vi "Test Harness.vi"() -> ()   [LabVIEW 2014, in "Waveform-Processing-Custom-Device Engine.lvlib"]
uses:
  Waveform-Processing-Custom-Device Engine.lvlib
  <vilib>/NI Veristand/Custom Device API/Hardware Interface Driver VI Operation.ctl
  <vilib>/NI Veristand/Custom Device API/Custom Device Item Ref.ctl
  <vilib>/NI Veristand/Custom Device API/Custom Device API.lvlib
panel:
  in  "Data Queue Element":dbl[](array[numeric])
  in  "Loop Rate":u32
  in  "Stop":bool
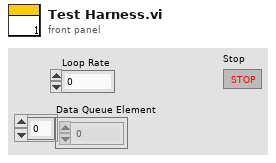
[diagram p1: front panel]
types:
  T1 = typedef "Custom Device API.lvlib/Hardware Interface Driver VI Operation.ctl" = enum16{"Initialize", "Start", "Read Data from HW", "Write Data to HW", "Close"}
  T2 = typedef "Custom Device API.lvlib/Custom Device Item Ref.ctl" = u64
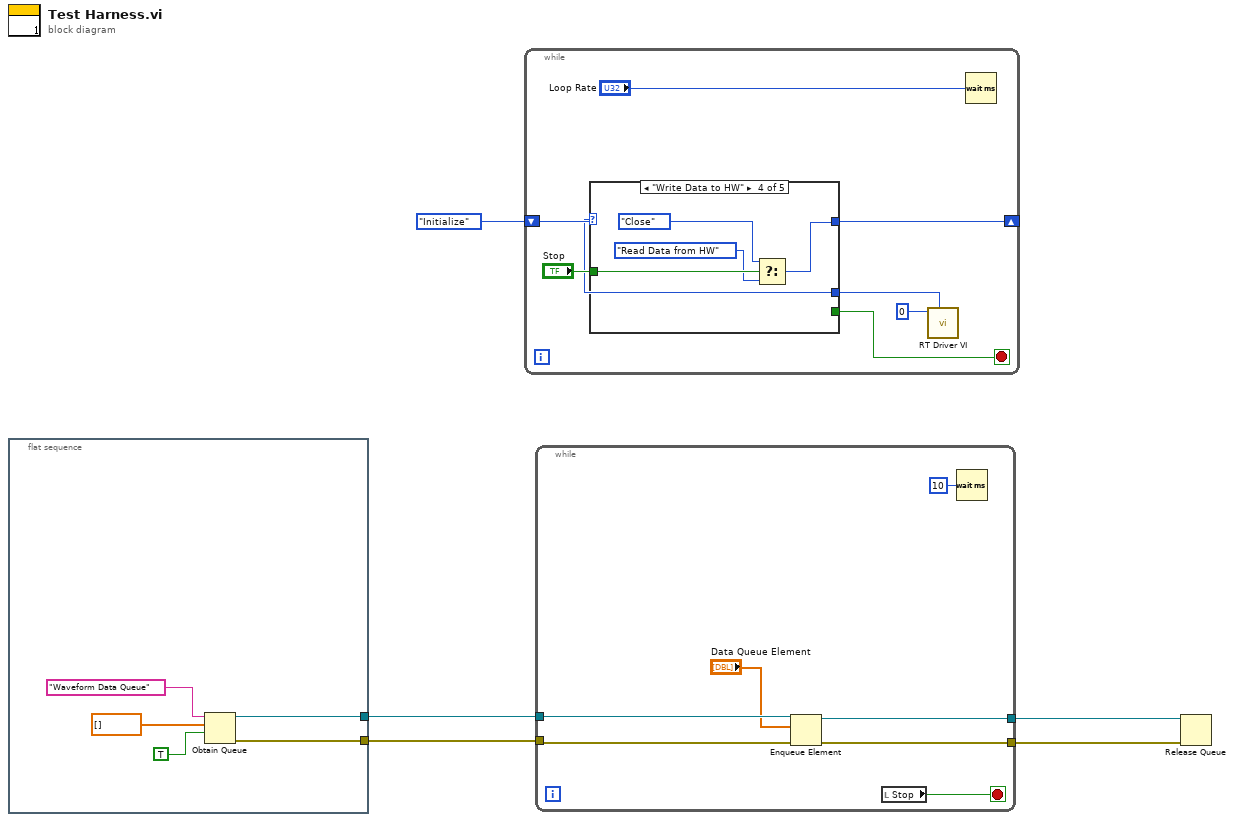
[diagram p0: block diagram]
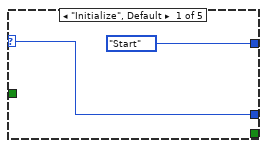
[diagram p2: hidden frame]
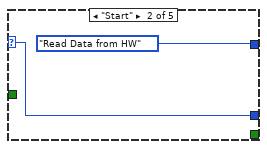
[diagram p3: hidden frame]
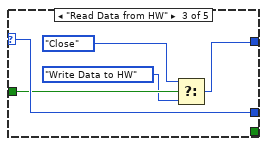
[diagram p4: hidden frame]
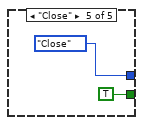
[diagram p5: hidden frame]
diagram:
  n1 = flat-sequence {
    tunnel: [w7] -> w3
    tunnel: [w6] -> w4
    frame #0 {
      n2 = Obtain Queue(name (unnamed)="Waveform Data Queue", element data type=dbl[] [], create if not found? (T)=TRUE) -> (queue out=w6:refnum<queue>, error out=w7:errorcluster)  [unwired: 2 in, 1 out]
    }
  }
  n3 = while {
    shift-right: [w15] -> _
    shift-left: Hardware_Interface_Driver_VI_Operation."Initialize" ("Operation") -> [w17]
    stop <- w13 stop-if-true
    n4 = case shown="\"Write Data to HW\"" w17 {
      selector: w17 -> [w19 w20 w26 w31 _]
      tunnel: [w19 w20 w26 w31 Hardware_Interface_Driver_VI_Operation."Close" ("Operation")] -> w16
      tunnel: [Hardware_Interface_Driver_VI_Operation."Start" ("Operation") Hardware_Interface_Driver_VI_Operation."Read Data from HW" ("Operation") w22 w27 _] -> w15
      tunnel: "Stop" -> [_ _ w25 w30 _]
      tunnel: [_ _ _ _ TRUE] -> w13
      frame "Initialize", Default {
      }
      frame "Start" {
      }
      frame "Read Data from HW" {
        n5 = Select(t=Hardware_Interface_Driver_VI_Operation."Close" ("Operation"), s=w25, f=Hardware_Interface_Driver_VI_Operation."Write Data to HW" ("Operation")) -> (s? t:f=w22:T1)
      }
      frame "Write Data to HW" {
        n6 = Select(t=Hardware_Interface_Driver_VI_Operation."Close" ("Operation"), s=w30, f=Hardware_Interface_Driver_VI_Operation."Read Data from HW" ("Operation")) -> (s? t:f=w27:T1)
      }
      frame "Close" {
      }
    }
    n7 = call "RT Driver VI.vi"("Operation"=w16, "Device Reference in"=T2 0) -> ()  [unwired: 9 in, 1 out]
    n8 = Wait (ms)(milliseconds to wait="Loop Rate") -> ()  [unwired: 1 out]
  }
  n9 = while {
    tunnel: w4 -> [w39]
    tunnel: w3 -> [w38]
    tunnel: [w37] -> w2
    tunnel: [w35] -> w1
    stop <- w40 stop-if-true
    n10 = Enqueue Element(queue=w39, element="Data Queue Element", error in (no error)=w38) -> (queue out=w35:refnum<queue>, error out=w37:errorcluster)  [unwired: 1 in, 1 out]
    n11 = local read "Stop"() -> (w40:bool)
    n12 = Wait (ms)(milliseconds to wait=u32 10) -> ()  [unwired: 1 out]
  }
  n13 = Release Queue(queue=w1, error in (no error)=w2) -> ()  [unwired: 1 in, 3 out]
